vi "Test QR Code Detector.vi"(11 "Test Case In":refnum<class "02_FeatureDetection.lvclass">) -> (0 "error out":errorcluster, 3 "Test Case Out":refnum<class "02_FeatureDetection.lvclass">)   [LabVIEW 2020, in "test.lvlib" / "02_FeatureDetection.lvclass"]
uses:
  02_FeatureDetection.lvclass
  02_FeatureDetection.lvclass/02_FeatureDetection.ctl
  4993e8ee-a06a-463a-9684-69129f64d5ce.vi
  feature_detection/WeChat QR Code Detector/WeChat QR Code Detector.lvclass
  aacecc5e-9590-4188-9100-b2fe39d53c4a.vi
  image/image.lvlib
  c620ff27-3bdc-43ee-ae28-79191c7efa9c.vi
  common/Image Point (Float).ctl
  common/common.lvlib
  feature_detection/WeChat QR Code Detector/Detection.ctl
  81cff08c-ad27-40c1-b34f-f5a0f1f6849e.vi
  common/Image Points Quad (Float).ctl
  feature_detection/WeChat QR Code Detector/Detect and Decode Multiple (ARGB).vi
  feature_detection/QR Code Encoder/QR Code Encoder.lvclass
  feature_detection/QR Code Encoder/Encode (Single).vi
  feature_detection/QR Code Encoder/Create (Single).vi
  image/New Image (ARGB Array).vi
  image/New Image (Greyscale Array).vi
  feature_detection/WeChat QR Code Detector/Detect and Decode Multiple (Greyscale).vi
  feature_detection/WeChat QR Code Detector/Create (Model Files Folder).vi
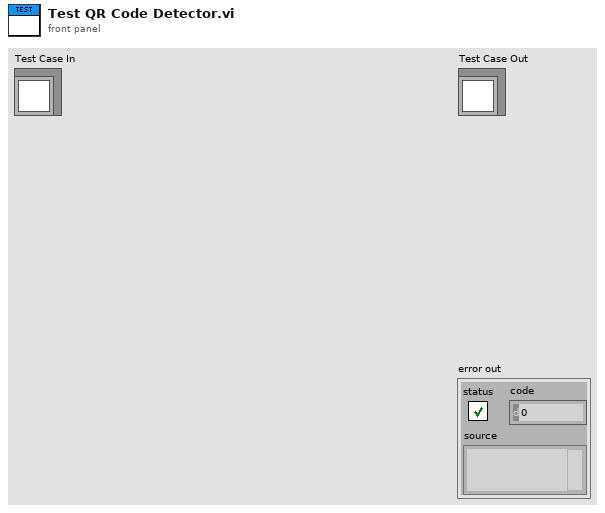
[diagram p1: front panel]
types:
  T1 = typedef "feature_detection.lvlib/WeChat QR Code Detector.lvclass/Detection.ctl" = cluster{"Data":string, "Corners":T2}
  T2 = typedef "common.lvlib/Image Points Quad (Float).ctl" = cluster{"A":T3, "B":T3, "C":T3, "D":T3}
  T3 = typedef "common.lvlib/Image Point (Float).ctl" = cluster{"x":dbl, "y":dbl}
  T4 = typedef "image.lvlib/ARGB Image.ctl" = refnum<data-value>
  T5 = typedef "image.lvlib/Greyscale Image.ctl" = refnum<data-value>
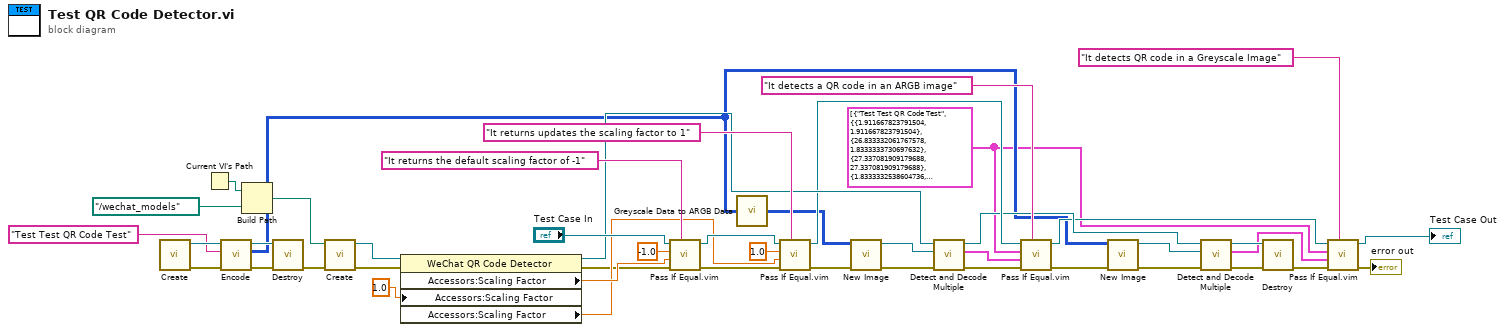
[diagram p0: block diagram]
diagram:
  w4 = T1[] [{"Data"="Test Test QR Code Test", "Corners"={"A"={"x"=1.911667823791504, "y"=1.911667823791504}, "B"={"x"=26.833332061767578, "y"=1.8333333730697632}, "C"={"x"=27.337081909179688, "y"=27.337081909179688}, "D"={"x"=1.8333332538604736, "y"=26.83333396911621}}}] ("Detections")
  n1 = call-poly "Create.vi"() -> ("error out"=w12:errorcluster, "QR Code Encoder"=w14:refnum<class "QR Code Encoder.lvclass">)  [unwired: 10 in]
  n2 = Current VI's Path() -> (path=w1:path)
  n3 = call-poly "Encode.vi"("error in (no error)"=w12, "Data"="Test Test QR Code Test", "QR Code Encoder in"=w14) -> ("error out"=w11:errorcluster, "QR Code Image Data"=w6:u8[][], "QR Code Encoder"=w13:refnum<class "QR Code Encoder.lvclass">)  [unwired: 6 in]
  n4 = Build Path(base path=w1, name or relative path=path "../wechat_models") -> (appended path=w2:path)
  n5 = call "Destroy.vi"("error in (no error)"=w11, "QR Code Encoder in"=w13) -> ("error out"=w9:errorcluster)  [unwired: 9 in]
  n6 = call-poly "Create.vi"("error in (no error)"=w9, "Model Files Directory"=w2) -> ("error out"=w42:errorcluster, "WeChat QR Code Detector"=w44:refnum<class "WeChat QR Code Detector.lvclass">)  [unwired: 8 in]
  n7 = property class="WeChat QR Code Detector"(reference=w44, error in=w42, "Accessors:Scaling Factor"=sgl 1.0 ("Scaling Factor")) -> (reference out=w32:refnum<class "WeChat QR Code Detector.lvclass">, error out=w34:errorcluster, "Accessors:Scaling Factor"=w41:sgl, "Accessors:Scaling Factor"=w35:sgl)
  n8 = call "Pass If Equal.vim"("Description"="It returns the default scaling factor of -1", "error in (no error)"=w34, "Actual"=w41, "Expected"=sgl -1.0 ("Scaling Factor"), "LUnit Test Case In"="Test Case In") -> ("error out"=w37:errorcluster, "LUnit Test Case Out"=w38:refnum<class "02_FeatureDetection.lvclass">)  [unwired: 5 in]
  n9 = call "Greyscale Data to ARGB Data.vi"("Greyscale Data"=w6) -> ("ARGB Data"=w8:u32[][])
  n10 = call "Pass If Equal.vim"("Description"="It returns updates the scaling factor to 1", "error in (no error)"=w37, "Actual"=w35, "Expected"=sgl 1.0 ("Scaling Factor"), "LUnit Test Case In"=w38) -> ("error out"=w31:errorcluster, "LUnit Test Case Out"=w29:refnum<class "02_FeatureDetection.lvclass">)  [unwired: 5 in]
  n11 = call-poly "New Image.vi"("error in (no error)"=w31, "U32 ARBG Data"=w8) -> ("error out"=w30:errorcluster, "ARGB Image"=w7:T4)  [unwired: 8 in]
  n12 = call-poly "Detect and Decode Multiple.vi"("error in (no error)"=w30, "ARGB Image in"=w7, "WeChat QR Code Detector in"=w32) -> ("error out"=w22:errorcluster, "Detections"=w5:T1[], "WeChat QR Code Detector"=w25:refnum<class "WeChat QR Code Detector.lvclass">)  [unwired: 6 in]
  n13 = call "Pass If Equal.vim"("Description"="It detects a QR code in an ARGB image", "error in (no error)"=w22, "Actual"=w5, "Expected"=w4, "LUnit Test Case In"=w29) -> ("error out"=w21:errorcluster, "LUnit Test Case Out"=w20:refnum<class "02_FeatureDetection.lvclass">)  [unwired: 5 in]
  n14 = call-poly "New Image.vi"("error in (no error)"=w21, "U8 Greyscale Data"=w6) -> ("error out"=w27:errorcluster, "Greyscale Image"=w26:T5)  [unwired: 8 in]
  n15 = call-poly "Detect and Decode Multiple.vi"("error in (no error)"=w27, "Greyscale Image in"=w26, "WeChat QR Code Detector in"=w25) -> ("error out"=w24:errorcluster, "Detections"=w15:T1[], "WeChat QR Code Detector"=w23:refnum<class "WeChat QR Code Detector.lvclass">)  [unwired: 6 in]
  n16 = call "Destroy.vi"("error in (no error)"=w24, "WeChat QR Code Detector in"=w23) -> ("error out"=w18:errorcluster)  [unwired: 9 in]
  n17 = call "Pass If Equal.vim"("Description"="It detects QR code in a Greyscale Image", "error in (no error)"=w18, "Actual"=w15, "Expected"=w4, "LUnit Test Case In"=w20) -> ("error out"=→"error out":errorcluster, "LUnit Test Case Out"=→"Test Case Out":refnum<class "02_FeatureDetection.lvclass">)  [unwired: 5 in]
